vi "shutdown endpoint.vi"(8 "error in":errorcluster, 10 "endpoint":i32, 11 "socket":i64) -> (0 "error out":errorcluster)   [LabVIEW 2013, in "lvnano.lvlib"]
doc: "NN_EXPORT int nn_shutdown (int s, int how);"
uses:
  lvnano.lvlib
  get last error code.vi
  get error string from code.vi
  <vilib>/Utility/error.llb/Error Cluster From Error Code.vi
  lvnanomsg.dll
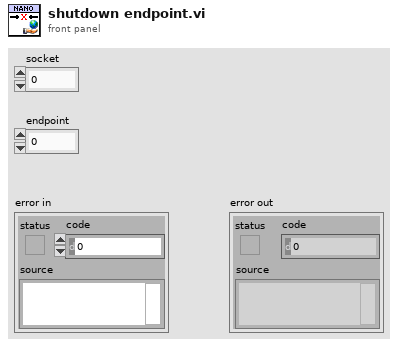
[diagram p1: front panel]
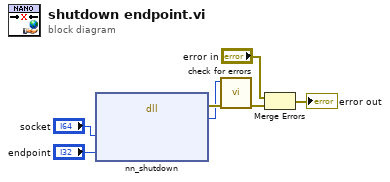
[diagram p0: block diagram]
diagram:
  n1 = dll-call lib="C:/Users/Daniel/Documents/nanomsg/lvnano/lvnanomsg.*" fn="nn_shutdown"("socket"="socket", "endpoint"="endpoint") -> (error out=w5:errorcluster, "error"=w3:i32)  [unwired: 5 in, 1 out]
  n2 = call "check for errors.vi"("error in"=w5, "function return"=w3) -> ("error out"=w4:errorcluster)  [unwired: 9 in]
  n3 = Merge Errors("error in", w4) -> (→"error out":errorcluster)
